vi "Read Rx from PLC.vi"(8 "error in (no error)":errorcluster, 11 "OPC UA in":refnum<class "OPC UA.lvclass">) -> (0 "error out":errorcluster, 2 "Rx from PLC":refnum<vi>, 3 "OPC UA out":refnum<class "OPC UA.lvclass">)   [LabVIEW 2019, in "OPC UA.lvlib" / "OPC UA.lvclass"]
uses:
  OPC UA.lvclass
  Tester Rx Dataset.ctl
  OPC UA.lvclass/OPC UA.ctl
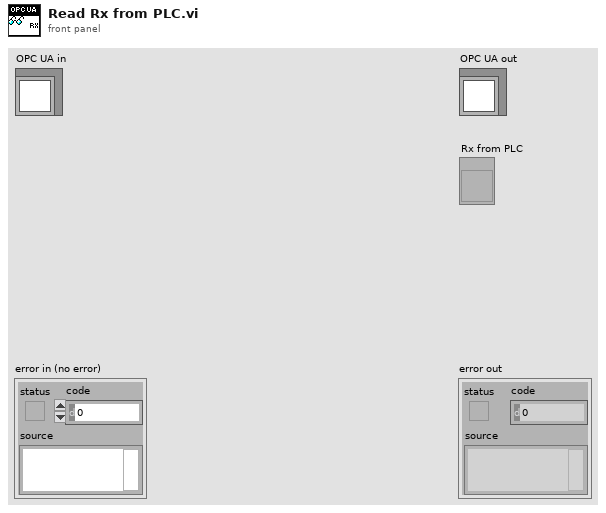
[diagram p1: front panel]
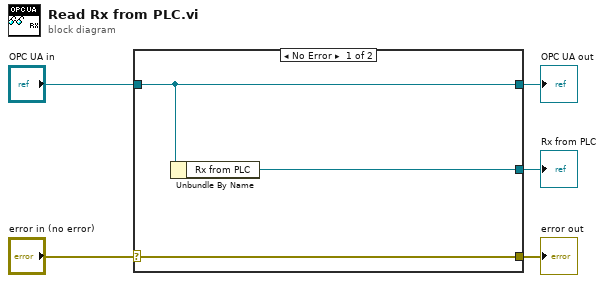
[diagram p0: block diagram]
diagram:
  n1 = case shown="No Error" "error in (no error)" {
    selector: "error in (no error)" -> [w8 w9]
    tunnel: [w8 w9] -> w4
    tunnel: [w7 w10] -> w2
    tunnel: "OPC UA in" -> [w7 w10]
    tunnel: [w6 _] -> w1
    frame No Error {
      n2 = Unbundle By Name(w7) -> ("Rx from PLC"=w6:refnum<vi>)
    }
    frame Error {
    }
  }
  "error out" <- w4
  "OPC UA out" <- w2
  "Rx from PLC" <- w1
